vi "ViewerUI.vi"() -> ()   [LabVIEW 2023]
uses:
  TypeDefs/ReceiverQueueOperations.ctl
  TypeDefs/ReceiverStateDataCluster.ctl
  TypeDefs/ReceiverDataCluster.ctl
  Classes/Communication/Communication.lvclass
  Classes/Receiver/Receiver.lvclass
  Classes/Sender/SenderUI.vi
  Classes/Receiver/ReceiverUI.vi
  Classes/Sender/Sender.lvclass
panel:
  in  "Run Sender":bool
  in  "Load Receiver":bool
  in  "Load Sender":bool
  out "error out":errorcluster
  in  "error in (no error)":errorcluster
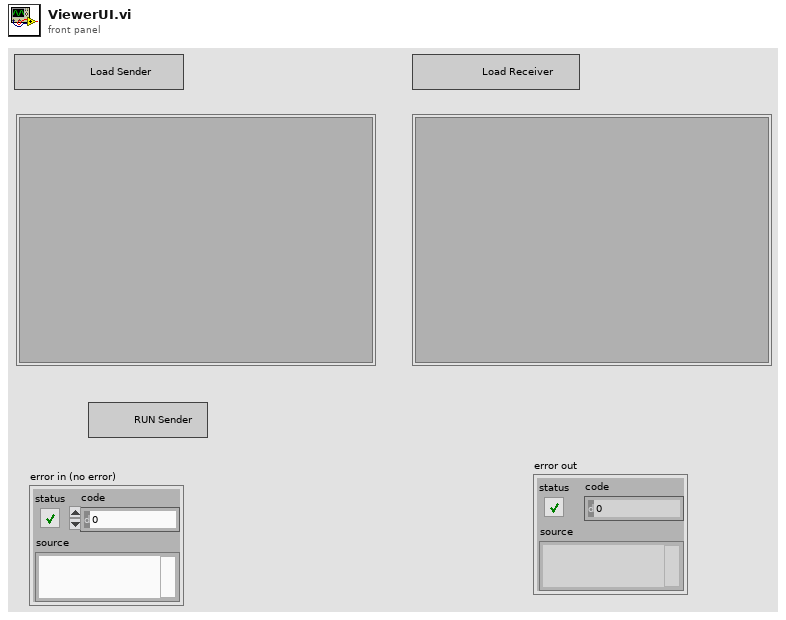
[diagram p1: front panel]
types:
  T1 = typedef "ReceiverDataCluster.ctl" = cluster{"Received Data":variant, "Communicate Class":refnum<class "Communication.lvclass">, "Load Sender":bool, "Load Receiver":bool, "Run Sender":bool, "Receiver Class":refnum<class "Receiver.lvclass">, "Message Status":bool}
  T2 = typedef "ReceiverStateDataCluster.ctl" = cluster{"State":string, "Data":variant}
  T3 = typedef "ReceiverQueueOperations.ctl" = enum16{"Init", "Enqueue", "Dequeue", "Enqueue N", "Flush", "Close", "Enqueue N Stack"}
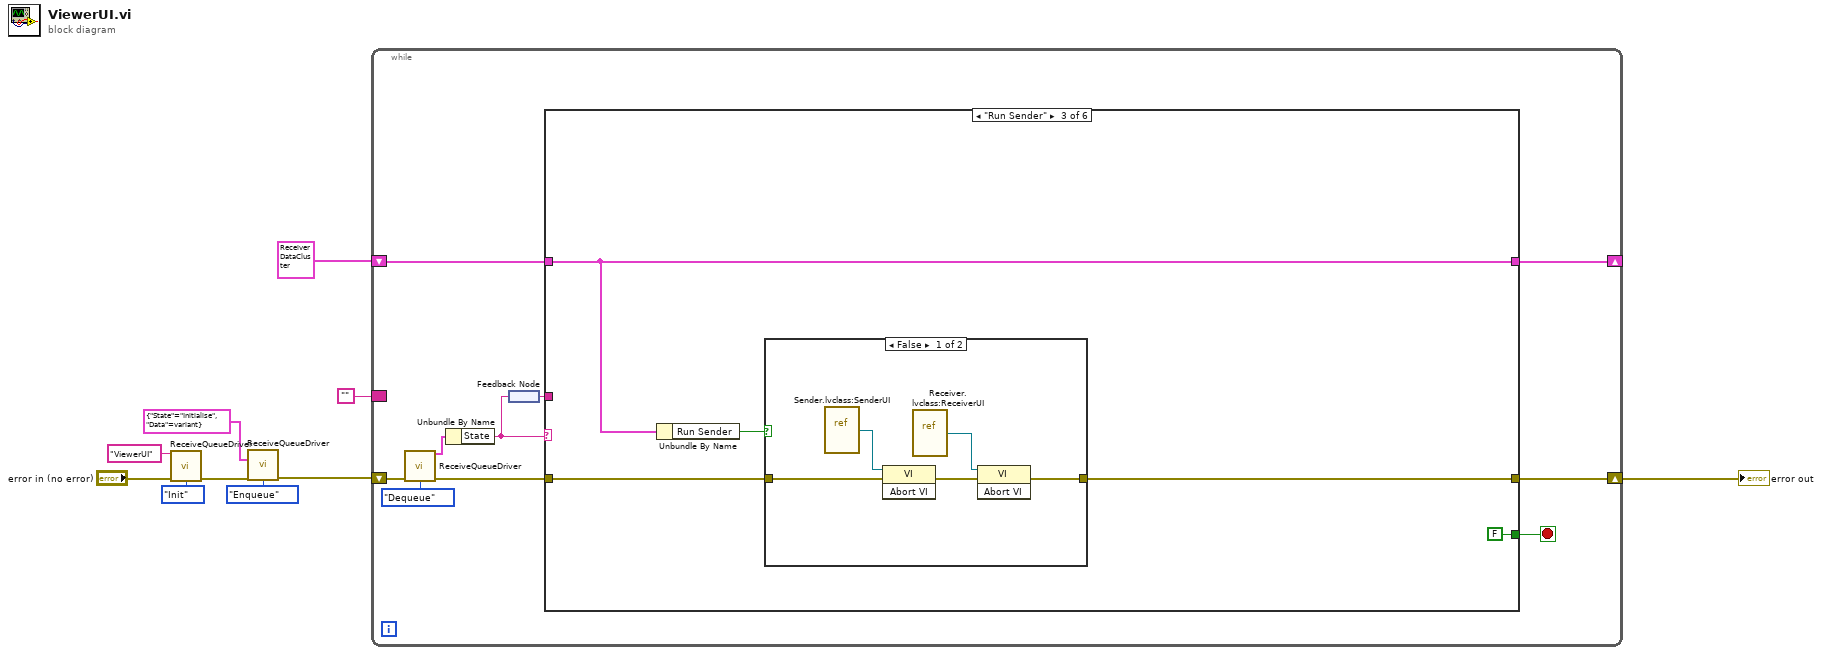
[diagram p0: block diagram]
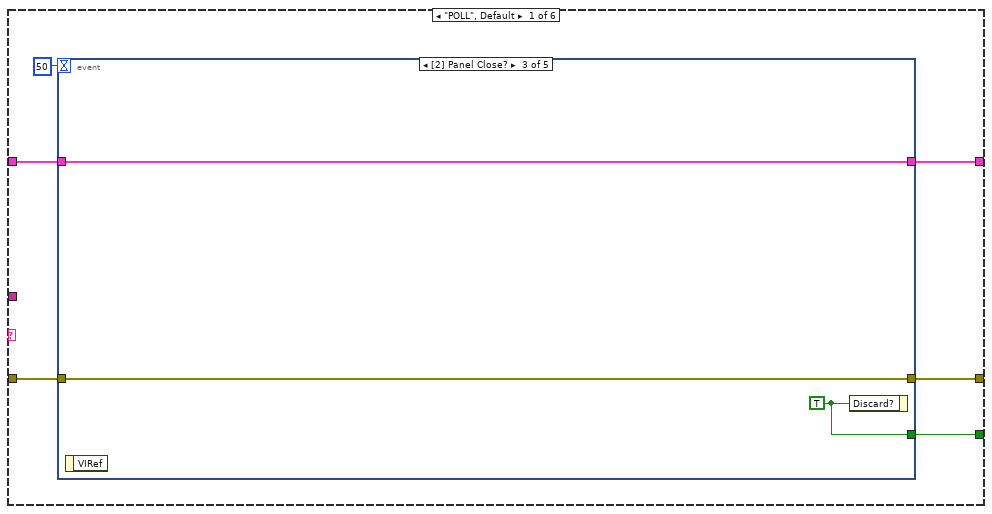
[diagram p2: hidden frame]
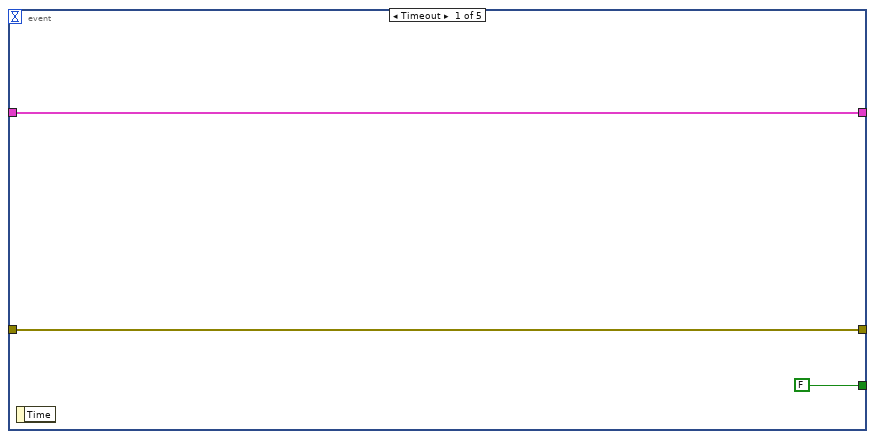
[diagram p3: hidden frame]
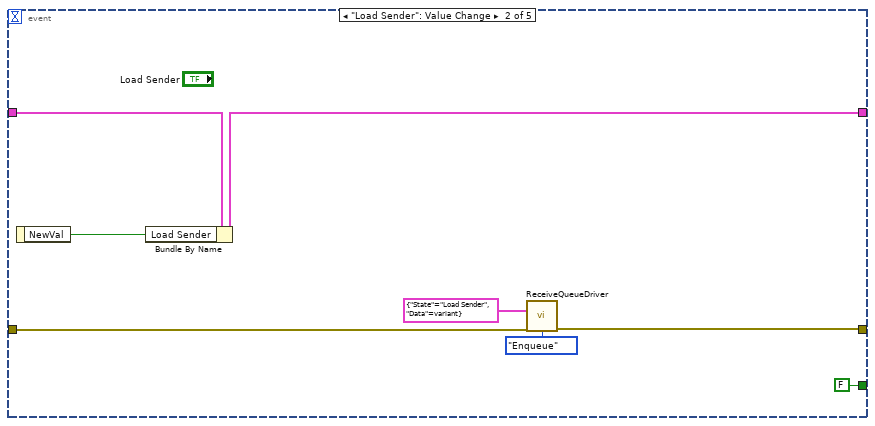
[diagram p4: hidden frame]
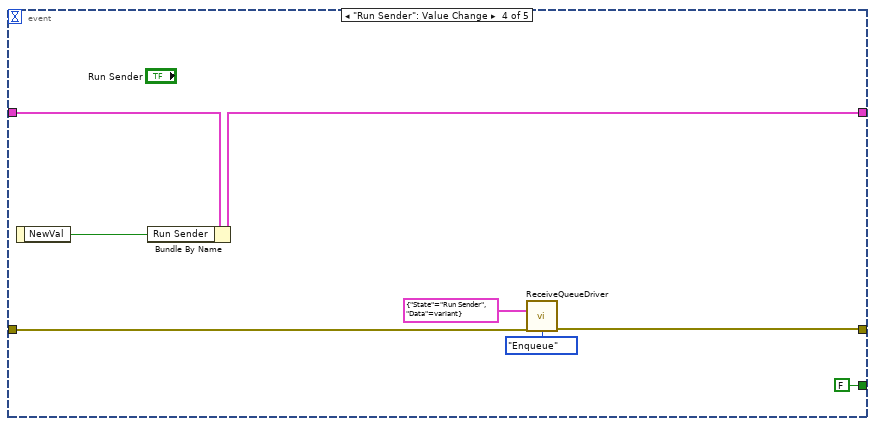
[diagram p5: hidden frame]
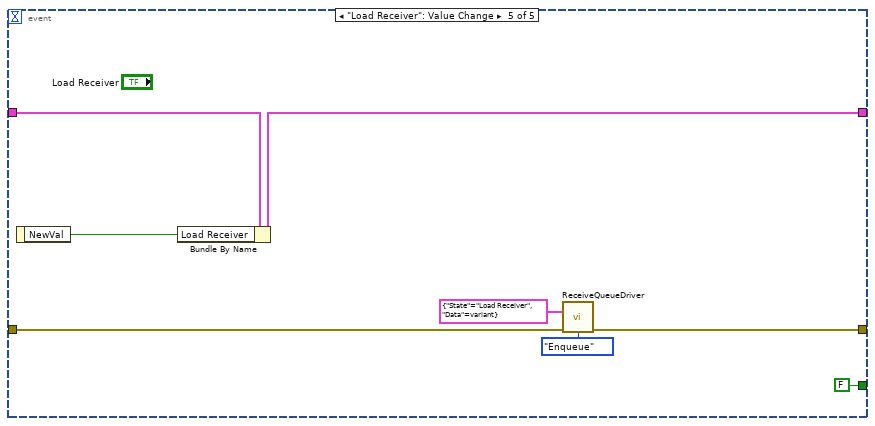
[diagram p6: hidden frame]
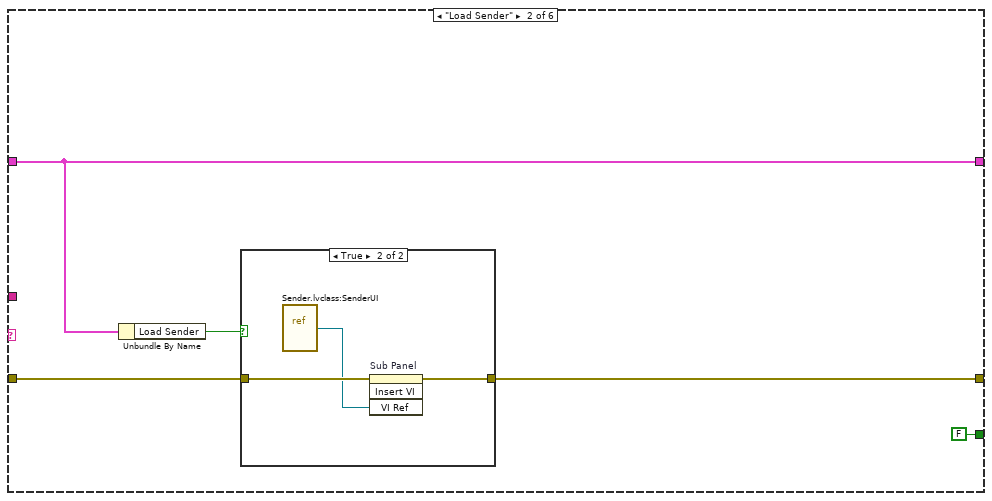
[diagram p7: hidden frame]
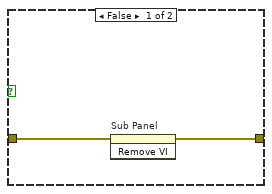
[diagram p8: hidden frame]
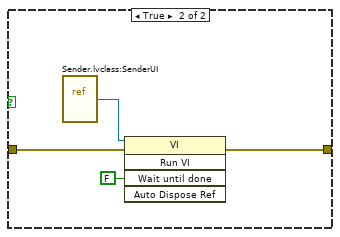
[diagram p9: hidden frame]
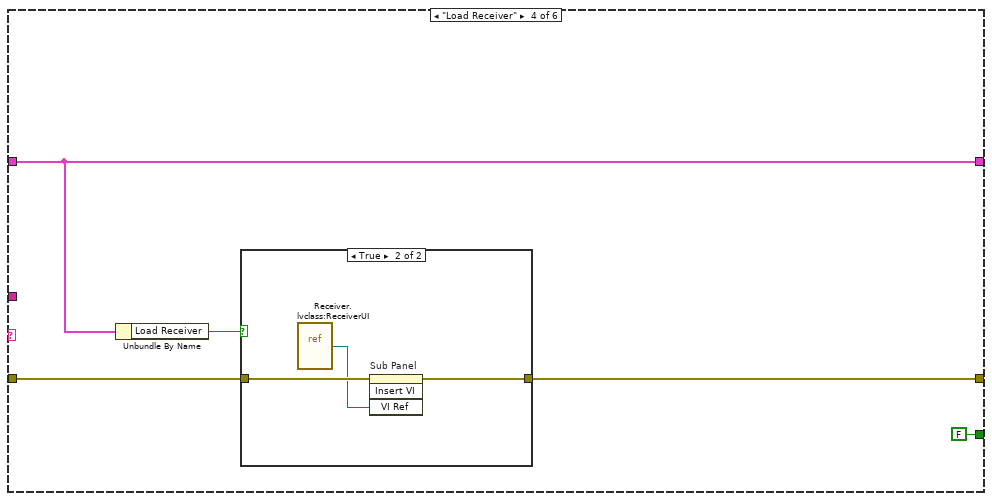
[diagram p10: hidden frame]
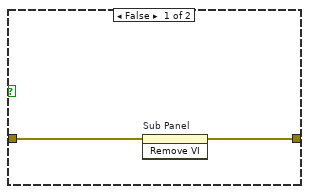
[diagram p11: hidden frame]
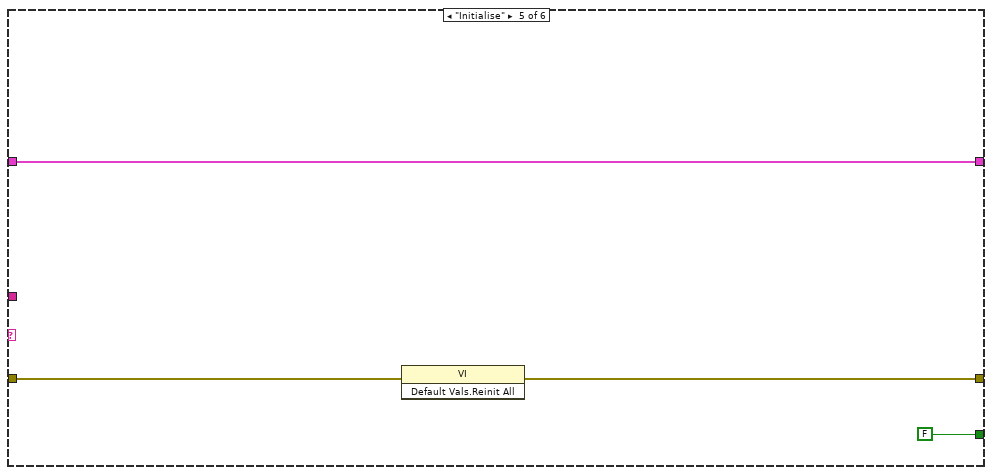
[diagram p12: hidden frame]
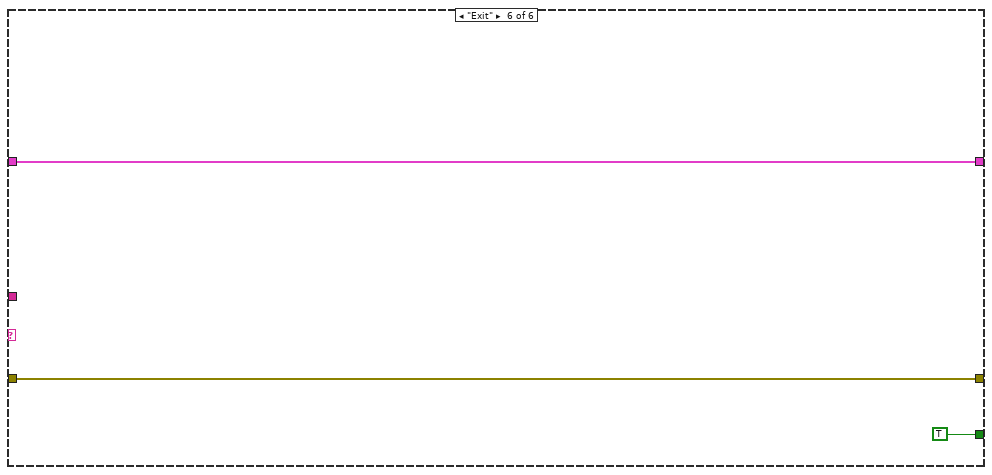
[diagram p13: hidden frame]
diagram:
  n1 = call "ReceiveQueueDriver.vi"("Queue Name"="ViewerUI", "error in (no error)"="error in (no error)", "Enum"=ReceiverQueueOperations."Init") -> ("error out"=w8:errorcluster)  [unwired: 11 in, 1 out]
  n2 = call "ReceiveQueueDriver.vi"("Enqueue Element"=T2 {"State"="Initialise", "Data"=variant}, "error in (no error)"=w8, "Enum"=ReceiverQueueOperations."Enqueue") -> ("error out"=w1:errorcluster)  [unwired: 11 in, 1 out]
  n3 = while {
    shift-right: [w20] -> w10
    shift-left: w1 -> [w19]
    shift-right: [w12] -> _
    shift-left: T1 {"Received Data"=variant, "Communicate Class"=refnum, "Load Sender"=FALSE, "Load Receiver"=FALSE, "Run Sender"=FALSE, "Receiver Class"=refnum, "Message Status"=FALSE} -> [w13]
    border: "" -> [_]
    stop <- w16 stop-if-true
    n4 = call "ReceiveQueueDriver.vi"("error in (no error)"=w19, "Enum"=ReceiverQueueOperations."Dequeue") -> ("Dequeue Element"=w17:T2, "error out"=w18:errorcluster)  [unwired: 12 in]
    n5 = Unbundle By Name(w17) -> ("State"=w15:string)
    n6 = feedback-in #1(w15) -> ()
    n7 = feedback #1() -> (w14:string)
    n8 = case shown="\"Run Sender\"" w15 {
      tunnel: w18 -> [w25 w60 w70 w84 w92 w96]
      tunnel: [w24 w59 w69 w83 w91 w96] -> w20
      tunnel: [w26 FALSE FALSE FALSE FALSE TRUE] -> w16
      tunnel: w14 -> [_ _ _ _ _ _]
      tunnel: w13 -> [w22 w58 w68 w82 w93 w97]
      tunnel: [w21 w58 w68 w82 w93 w97] -> w12
      frame "POLL", Default {
        n9 = event shown="[2] Panel Close?" {
          selector: _ -> [_ _ _ _ _]
          dyn-events: _ -> [_ _ _ _ _]
          timeout: 50 -> [_ _ _ _ _]
          tunnel: [FALSE FALSE w39 FALSE FALSE] -> w26
          tunnel: w25 -> [w28 w32 w38 w43 w50]
          tunnel: [w28 w31 w38 w42 w49] -> w24
          tunnel: w22 -> [w27 w37 w40 w48 w56]
          tunnel: [w27 w35 w40 w46 w54] -> w21
          event Timeout {
            n10 = event-data() -> ()  [unwired: 1 in, 1 out]
          }
          event "Load Sender": Value Change {
            n11 = event-data() -> ("NewVal"=w34:bool)  [unwired: 1 in]
            n12 = Bundle By Name(cluster=w37, "Load Sender"=w34) -> (w35:T1)
            n13 = call "ReceiveQueueDriver.vi"("Enqueue Element"=T2 {"State"="Load Sender", "Data"=variant}, "error in (no error)"=w32, "Enum"=ReceiverQueueOperations."Enqueue") -> ("error out"=w31:errorcluster)  [unwired: 11 in, 1 out]
          }
          event Panel Close? {
            w39 = TRUE ("Discard?")
            n14 = event-data() -> ()  [unwired: 1 in, 1 out]
            n15 = event-data("Discard?"=w39) -> ()  [unwired: 1 in, 1 out]
          }
          event "Run Sender": Value Change {
            n16 = event-data() -> ("NewVal"=w45:bool)  [unwired: 1 in]
            n17 = Bundle By Name(cluster=w48, "Run Sender"=w45) -> (w46:T1)
            n18 = call "ReceiveQueueDriver.vi"("Enqueue Element"=T2 {"State"="Run Sender", "Data"=variant}, "error in (no error)"=w43, "Enum"=ReceiverQueueOperations."Enqueue") -> ("error out"=w42:errorcluster)  [unwired: 11 in, 1 out]
          }
          event "Load Receiver": Value Change {
            n19 = event-data() -> ("NewVal"=w53:bool)  [unwired: 1 in]
            n20 = Bundle By Name(cluster=w56, "Load Receiver"=w53) -> (w54:T1)
            n21 = call "ReceiveQueueDriver.vi"("Enqueue Element"=T2 {"State"="Load Receiver", "Data"=variant}, "error in (no error)"=w50, "Enum"=ReceiverQueueOperations."Enqueue") -> ("error out"=w49:errorcluster)  [unwired: 11 in, 1 out]
          }
        }
      }
      frame "Load Sender" {
        n22 = Unbundle By Name(w58) -> ("Load Sender"=w57:bool)
        n23 = case shown="True" w57 {
          tunnel: w60 -> [w63 w66]
          tunnel: [w62 w65] -> w59
          frame False {
            n24 = invoke on="Sub Panel" class="SubPnl" method="Remove VI"(error in=w63) -> (error out=w62:errorcluster)  [unwired: 2 in, 2 out]
          }
          frame True {
            n25 = vi-ref "Sender.lvclass:SenderUI.vi"() -> (w64:refnum<vi>)
            n26 = invoke on="Sub Panel" class="SubPnl" method="Insert VI"(error in=w66, "VI Ref"=w64) -> (error out=w65:errorcluster)  [unwired: 2 in, 3 out]
          }
        }
      }
      frame "Run Sender" {
        n27 = Unbundle By Name(w68) -> ("Run Sender"=w67:bool)
        n28 = case shown="False" w67 {
          tunnel: w70 -> [w76 w80]
          tunnel: [w73 w79] -> w69
          frame False {
            n29 = vi-ref "Sender.lvclass:SenderUI.vi"() -> (w75:refnum<vi>)
            n30 = invoke class="VI" method="Abort VI"(reference=w75, error in=w76) -> (error out=w74:errorcluster)  [unwired: 1 in, 2 out]
            n31 = vi-ref "Receiver.lvclass:ReceiverUI.vi"() -> (w72:refnum<vi>)
            n32 = invoke class="VI" method="Abort VI"(reference=w72, error in=w74) -> (error out=w73:errorcluster)  [unwired: 1 in, 2 out]
          }
          frame True {
            n33 = vi-ref "Sender.lvclass:SenderUI.vi"() -> (w78:refnum<vi>)
            n34 = invoke class="VI" method="Run VI"(reference=w78, error in=w80, "Wait until done"=FALSE ("Wait Until Done")) -> (error out=w79:errorcluster)  [unwired: 2 in, 4 out]
          }
        }
      }
      frame "Load Receiver" {
        n35 = Unbundle By Name(w82) -> ("Load Receiver"=w81:bool)
        n36 = case shown="True" w81 {
          tunnel: w84 -> [w87 w90]
          tunnel: [w86 w89] -> w83
          frame False {
            n37 = invoke on="Sub Panel" class="SubPnl" method="Remove VI"(error in=w87) -> (error out=w86:errorcluster)  [unwired: 2 in, 2 out]
          }
          frame True {
            n38 = vi-ref "Receiver.lvclass:ReceiverUI.vi"() -> (w88:refnum<vi>)
            n39 = invoke on="Sub Panel" class="SubPnl" method="Insert VI"(error in=w90, "VI Ref"=w88) -> (error out=w89:errorcluster)  [unwired: 2 in, 3 out]
          }
        }
      }
      frame "Initialise" {
        n40 = invoke class="VI" method="Default Vals.Reinit All"(error in=w92) -> (error out=w91:errorcluster)  [unwired: 2 in, 2 out]
      }
      frame "Exit" {
      }
    }
  }
  "error out" <- w10
